vi "Set TriggerLevel.vi"(8 "error in (no error)":errorcluster, 9 "Valid String?":bool, 10 "Trigger Value":string, 11 "VISA Refnum in":refnum<visa-resource-name>) -> (0 "error out":errorcluster, 1 "Array of Strings 2":string[](array[string]), 2 "Energy Mode OFF ACK?":string="\r\n", 3 "triggervalue ACK?":string, 4 "Energy ON ACK?":string="\r\r\n", 5 "Trig Level":dbl, 7 "Array of Strings 4":string[](array[string]))   [LabVIEW 2013, in "Gentec Plink.lvclass"]
uses:
  Gentec Plink.lvclass
  Serial Commands.ctl
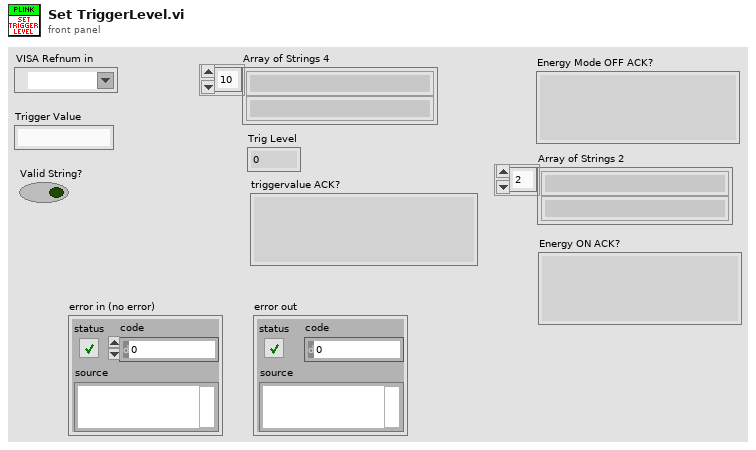
[diagram p1: front panel]
types:
  T1 = typedef "OnOffTypeDef.ctl" = enum16{"off", "on"}
  T2 = typedef "Serial Commands.ctl" = i32
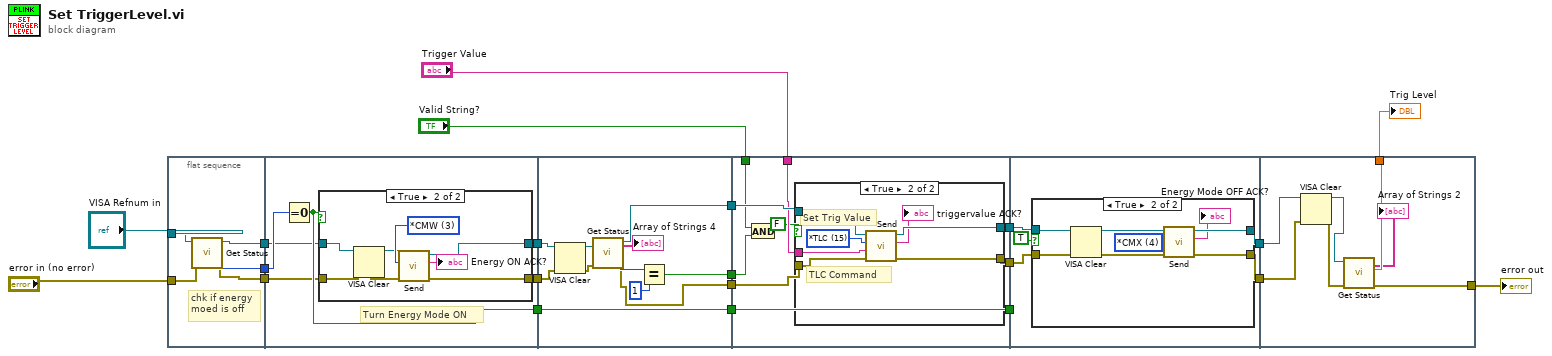
[diagram p0: block diagram]
diagram:
  n1 = flat-sequence {
    tunnel: "VISA Refnum in" -> [w26]
    tunnel: "error in (no error)" -> [w25]
    tunnel: [w24] -> w21
    tunnel: [w23] -> w20
    tunnel: [w22] -> w19
    tunnel: w21 -> [w32]
    tunnel: [w31] -> w18
    tunnel: w20 -> [w30]
    tunnel: [w29] -> w17
    tunnel: w19 -> [w28]
    tunnel: [w27] -> w16
    tunnel: w18 -> [w53]
    tunnel: [w53] -> w15
    tunnel: w17 -> [w52]
    tunnel: [w49] -> w14
    tunnel: [w48] -> w13
    tunnel: w16 -> [w45]
    tunnel: [w47] -> w12
    tunnel: [w62] -> w11
    tunnel: w15 -> [w62]
    tunnel: w14 -> [w56]
    tunnel: w13 -> [w61]
    tunnel: [w60] -> w10
    tunnel: w12 -> [w59]
    tunnel: [w58] -> w9
    tunnel: "Valid String?" -> [w57]
    tunnel: "Trigger Value" -> [w55]
    tunnel: w11 -> [_]
    tunnel: w10 -> [w76]
    tunnel: [w75] -> w8
    tunnel: w9 -> [w74]
    tunnel: [w73] -> w7
    tunnel: w8 -> [w90]
    tunnel: [w93] -> w5
    tunnel: w7 -> [w89]
    tunnel: [w92] -> w3
    frame #0 {
      # "chk if energy\nmoed is off"
      n2 = call "Get Status.vi"("error in (no error)"=w25, "ConnectionIn"=w26) -> ("error out"=w22:errorcluster, "Energy Mode"=w24:T1, "VISA Refnum out"=w23:refnum<visa-resource-name>)  [unwired: 3 in, 4 out]
    }
    frame #1 {
      # "Turn Energy Mode ON"
      n3 = Equal To 0?(x=w32) -> (x = 0?=w31:bool)
      n4 = case shown="True" w31 {
        tunnel: w30 -> [w34 w41]
        tunnel: [w34 w40] -> w29
        tunnel: w28 -> [w33 w37]
        tunnel: [w33 w39] -> w27
        frame False {
        }
        frame True {
          w42 = T2 3 items=["*CAU", "*RST", "*KPA", "*CMW", "*CMX", "*F01", "*SHI", "*CSU", "*SLO", "*MUL", "*FAS", "*CFF", "*CFT", "*OFF"] ("string to write")
          n5 = VISA Clear(VISA resource name=w41, error in (no error)=w37) -> (VISA resource name out=w38:refnum<visa-resource-name>, error out=w36:errorcluster)
          n6 = call "Send.vi"("error in (no error)"=w36, "Command"=w42, "VISA Refnum in"=w38) -> ("error out"=w39:errorcluster, "read buffer"=→"Energy ON ACK?":string, "VISA Refnum out"=w40:refnum<visa-resource-name>)  [unwired: 6 in]
        }
      }
    }
    frame #2 {
      n7 = VISA Clear(VISA resource name=w52, error in (no error)=w45) -> (VISA resource name out=w46:refnum<visa-resource-name>, error out=w44:errorcluster)
      n8 = call "Get Status.vi"("error in (no error)"=w44, "ConnectionIn"=w46) -> ("error out"=w47:errorcluster, "Energy Mode"=w51:T1, "VISA Refnum out"=w48:refnum<visa-resource-name>, "Array of Strings"=→"Array of Strings 4":string[])  [unwired: 3 in, 3 out]
      n9 = Equal?(x=w51, y=1) -> (x = y?=w49:bool)
    }
    frame #3 {
      n10 = And(x=w57, y=w56) -> ()  [unwired: 1 out]
      n11 = case shown="True" FALSE {
        tunnel: w61 -> [w64 w70]
        tunnel: [w64 w69] -> w60
        tunnel: w59 -> [w63 w68]
        tunnel: [w63 w67] -> w58
        tunnel: w55 -> [_ w66]
        frame False {
        }
        frame True {
          w71 = T2 15 items=["*CAU", "*RST", "*KPA", "*CMW", "*CMX", "*F01", "*SHI", "*CSU", "*SLO", "*MUL", "*FAS", "*CFF", "*CFT", "*CVU", "*OFF", "*TLC"] ("string to write")
          # "Set Trig Value"
          # "TLC Command"
          n12 = call "Send.vi"("error in (no error)"=w68, "Option"=w66, "Command"=w71, "VISA Refnum in"=w70) -> ("error out"=w67:errorcluster, "read buffer"=→"triggervalue ACK?":string, "VISA Refnum out"=w69:refnum<visa-resource-name>)  [unwired: 5 in]
        }
      }
    }
    frame #4 {
      n13 = case shown="True" TRUE {
        tunnel: w76 -> [w78 w82]
        tunnel: [w78 w85] -> w75
        tunnel: w74 -> [w77 w83]
        tunnel: [w77 w84] -> w73
        frame False {
        }
        frame True {
          w86 = T2 4 items=["*CAU", "*RST", "*KPA", "*CMW", "*CMX", "*F01", "*SHI", "*CSU", "*SLO", "*MUL", "*FAS", "*CFF", "*CFT", "*OFF"] ("string to write")
          n14 = VISA Clear(VISA resource name=w82, error in (no error)=w83) -> (VISA resource name out=w81:refnum<visa-resource-name>, error out=w80:errorcluster)
          n15 = call "Send.vi"("error in (no error)"=w80, "Command"=w86, "VISA Refnum in"=w81) -> ("error out"=w84:errorcluster, "read buffer"=→"Energy Mode OFF ACK?":string, "VISA Refnum out"=w85:refnum<visa-resource-name>)  [unwired: 6 in]
        }
      }
    }
    frame #5 {
      n16 = VISA Clear(VISA resource name=w90, error in (no error)=w89) -> (VISA resource name out=w88:refnum<visa-resource-name>, error out=w87:errorcluster)
      n17 = call "Get Status.vi"("error in (no error)"=w87, "ConnectionIn"=w88) -> ("error out"=w92:errorcluster, "Trig Level"=w93:dbl, "Array of Strings"=→"Array of Strings 2":string[])  [unwired: 3 in, 4 out]
    }
  }
  "Trig Level" <- w5
  "error out" <- w3
